vi "Dynamic Bit Depth Encoding x1 (SubVI).vi"(0 "Pixel Data In":u8, 5 "Pixel In Valid?":bool=TRUE, 8 "Block Size x2":u16=8, 10 "Block Size":u16=8, 12 "Image Width":u16=512) -> (14 "Bit Depth":u8, 15 "Minimum":u8, 16 "Result Valid?":bool, 18 "Data Out":u8, 19 "Output Valid?":bool)   [LabVIEW 2014]
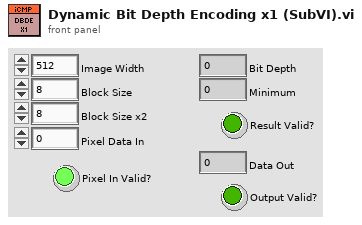
[diagram p1: front panel]
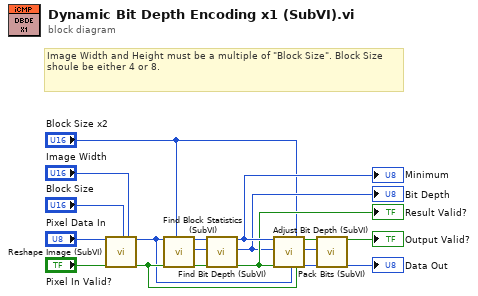
[diagram p0: block diagram]
diagram:
  # "Image Width and Height must be a multiple of \"Block Size\". Block Size shoule be either 4 or 8."
  n1 = call "Reshape Image (SubVI).vi"("Pixel Data In"="Pixel Data In", "Pixel In Valid?"="Pixel In Valid?", "Block Size"="Block Size", "Image Width"="Image Width") -> ("Pixel Data Out"=w8:u8, "Pixel Out Valid?"=w9:bool)  [unwired: 14 in]
  n2 = call "Find Block Statistics (SubVI).vi"("Pixel Data"=w8, "Pixel Valid?"=w9, "Block Size x2"="Block Size x2") -> ("Maximum"=w5:u8, "Minimum"=w6:u8, "Result Valid?"=w7:bool)  [unwired: 14 in]
  n3 = call "Find Bit Depth (SubVI).vi"("Maximum"=w5, "Minimum (In)"=w6, "Input Valid?"=w7) -> ("Minimum (Out)"=w13:u8, "Bit Depth"=w11:u8, "Output Valid?"=w12:bool)  [unwired: 14 in]
  "Result Valid?" <- w12
  "Minimum" <- w13
  "Bit Depth" <- w11
  n4 = call "Adjust Bit Depth (SubVI).vi"("Minimum"=w13, "Bit Depth"=w11, "Stat. Valid?"=w12, "Pixel Data"=w8, "Block Size x2"="Block Size x2", "Pixel Valid?"=w9) -> ("Output Valid?"=w4:bool, "Data Out"=w3:u8, "Bid Depth Out"=w2:u8)  [unwired: 11 in]
  n5 = call "Pack Bits (SubVI).vi"("Input Valid?"=w4, "Data In"=w3, "Bit Depth"=w2) -> ("Output Valid?"=→"Output Valid?":bool, "Data Out"=→"Data Out":u8)  [unwired: 15 in]
